vi "Cleanup Server.vi"(8 "error in (no error)":errorcluster, 11 "TCPMessaging in":refnum<class "TCPMessaging.lvclass">) -> (0 "error out":errorcluster)   [LabVIEW 2020, in "Vecto.lvlib" / "TCPMessaging.lvclass"]
uses:
  TCPMessaging.lvclass
  TCPMessaging.lvclass/TCPMessaging.ctl
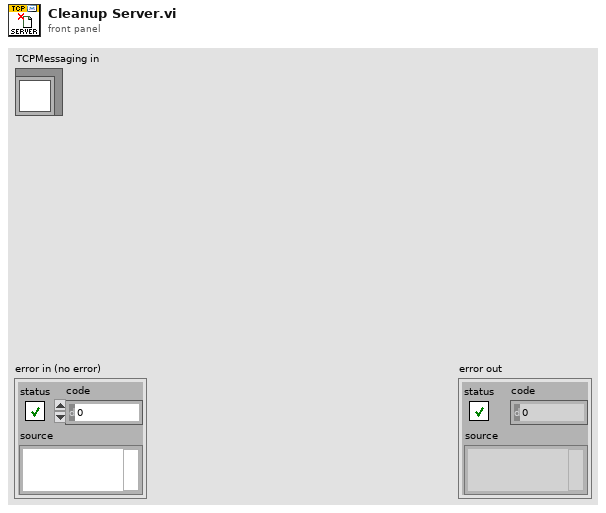
[diagram p1: front panel]
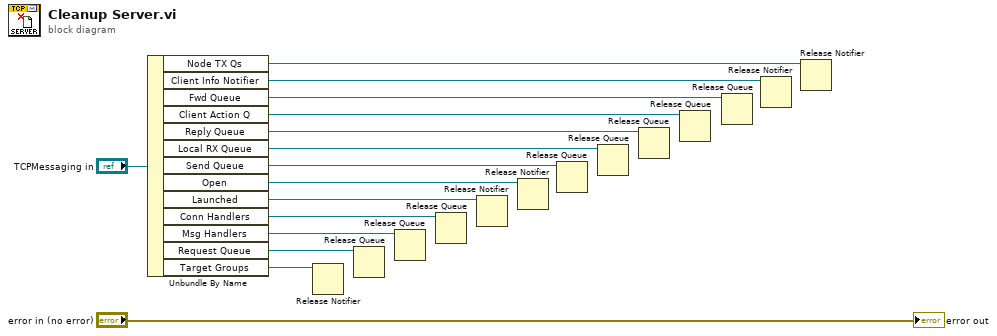
[diagram p0: block diagram]
diagram:
  n1 = Unbundle By Name("TCPMessaging in") -> ("Node TX Qs"=w1:refnum<notifier>, "Client Info Notifier"=w2:refnum<notifier>, "Fwd Queue"=w3:refnum<queue>, "Client Action Q"=w4:refnum<queue>, "Reply Queue"=w10:refnum<queue>, "Local RX Queue"=w11:refnum<queue>, "Send Queue"=w12:refnum<queue>, "Open"=w13:refnum<notifier>, "Launched"=w9:refnum<notifier>, "Conn Handlers"=w8:refnum<queue>, "Msg Handlers"=w7:refnum<queue>, "Request Queue"=w6:refnum<queue>, "Target Groups"=w5:refnum<notifier>)
  n2 = Release Notifier(notifier=w5) -> ()  [unwired: 2 in, 3 out]
  n3 = Release Queue(queue=w6) -> ()  [unwired: 2 in, 3 out]
  n4 = Release Queue(queue=w7) -> ()  [unwired: 2 in, 3 out]
  n5 = Release Queue(queue=w8) -> ()  [unwired: 2 in, 3 out]
  n6 = Release Notifier(notifier=w9) -> ()  [unwired: 2 in, 3 out]
  n7 = Release Notifier(notifier=w13) -> ()  [unwired: 2 in, 3 out]
  n8 = Release Queue(queue=w12) -> ()  [unwired: 2 in, 3 out]
  n9 = Release Queue(queue=w11) -> ()  [unwired: 2 in, 3 out]
  n10 = Release Queue(queue=w10) -> ()  [unwired: 2 in, 3 out]
  n11 = Release Queue(queue=w4) -> ()  [unwired: 2 in, 3 out]
  n12 = Release Queue(queue=w3) -> ()  [unwired: 2 in, 3 out]
  n13 = Release Notifier(notifier=w2) -> ()  [unwired: 2 in, 3 out]
  n14 = Release Notifier(notifier=w1) -> ()  [unwired: 2 in, 3 out]
  "error out" <- "error in (no error)"
